vi "Telnet Connection Destructor.vi"(0 "object data in":T1) -> ()   [LabVIEW 2015, in "NI_InternetTK_Core_VIs.lvlib"]
doc: "Function that cleans up when an object is destroyed.\nIt may close a file or connection, or may need to trigger an occurrence."
uses:
  NI_InternetTK_Core_VIs.lvlib
  Telnet Connection Data.ctl
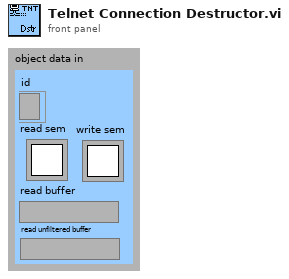
[diagram p1: front panel]
types:
  T1 = typedef "Telnet Connection Data.ctl" = cluster{"id":refnum<k5>, "read sem":T2, "write sem":T2, "read buffer":string, "read unfiltered buffer":string}
  T2 = typedef "__Semaphore RefNum" = refnum<k1>
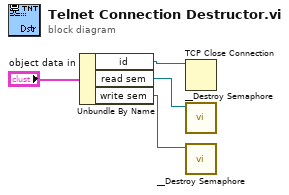
[diagram p0: block diagram]
diagram:
  n1 = Unbundle By Name("object data in") -> ("id"=w3:refnum<k5>, "read sem"=w2:T2, "write sem"=w1:T2)
  n2 = TCP Close Connection(connection ID=w3) -> ()  [unwired: 1 in, 3 out]
  n3 = call "__Destroy Semaphore.vi"("semaphore"=w2) -> ()  [unwired: 1 in, 6 out]
  n4 = call "__Destroy Semaphore.vi"("semaphore"=w1) -> ()  [unwired: 1 in, 6 out]
